vi "SubVI_HP4263A_1kHz.vi"(4 "error in (no error)":errorcluster, 5 "averaging count (1)":i16=1 min=1 max=256 step=1, 6 "function (Z - Angle:0)":u16(ring) items=["Z - Angle", "R - X", "Y - Angle", "G - B", "CP - D", "CP - Q", "CP - G", "CS - D", "CS - Q", "CS - RS", "LP - D", "LP - Q", "LP - G", "LS - D", "LS - Q", "LS - RS", "LS - DCR (option 001 only)", "LP - DCR (option 001 only)", "L2 - N (option 001 only)", "L2 - M (option 001 only)", "L2 - R2 (option 001 only)"], 7 "VISA resource name":refnum<visa-resource-name>) -> (0 "error out":errorcluster, 1 "secondary reading":dbl format="%.5e", 2 "primary reading":dbl format="%.5e", 3 "status":u16)   [LabVIEW 2010]
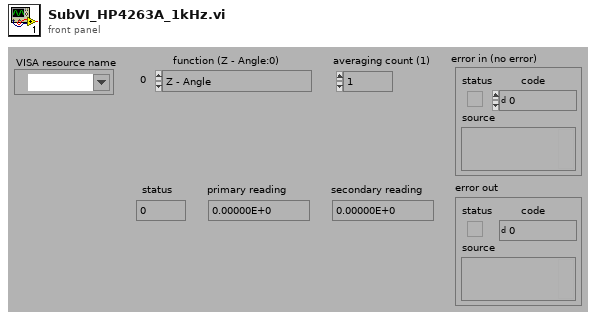
[diagram p1: front panel]
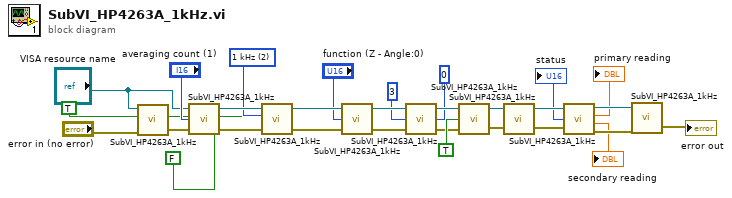
[diagram p0: block diagram]
diagram:
  w25 = u16 2 items=["100 Hz", "120 Hz", "1 kHz", "10 kHz", "20 kHz (option 002 ONLY)", "100 kHz"] ("frequency (100 Hz:0)")
  n1 = call "SubVI_HP4263A_1kHz.vi"("error in (no error)"="error in (no error)", "VISA resource name"="VISA resource name") -> ("error out"=w20:errorcluster)  [unwired: 2 in, 3 out]
  n2 = call "SubVI_HP4263A_1kHz.vi"("state (on:T)"=FALSE, "error in (no error)"=w20, "count (1)"="averaging count (1)", "VISA session"="VISA resource name") -> ("error out"=w28:errorcluster, "dup VISA session"=w26:refnum<visa-resource-name>)
  n3 = call "SubVI_HP4263A_1kHz.vi"("error in (no error)"=w28, "line frequency (60 Hz:F)"=TRUE, "frequency (100 Hz:0)"=w25, "VISA session"=w26) -> ("error out"=w29:errorcluster, "dup VISA session"=w27:refnum<visa-resource-name>)  [unwired: 1 in]
  n4 = call "SubVI_HP4263A_1kHz.vi"("error in (no error)"=w29, "function (Z - Angle:0)"="function (Z - Angle:0)", "VISA session"=w27) -> ("error out"=w9:errorcluster, "dup VISA session"=w8:refnum<visa-resource-name>)  [unwired: 1 in]
  n5 = call "SubVI_HP4263A_1kHz.vi"("trigger delay (sec)"=0, "error in (no error)"=w9, "trigger source (int:0)"=3, "VISA session"=w8) -> ("error out"=w13:errorcluster, "dup VISA session"=w14:refnum<visa-resource-name>)
  n6 = call "SubVI_HP4263A_1kHz.vi"("error in (no error)"=w13, "initiate mode (cont:T)"=TRUE, "VISA session"=w14) -> ("error out"=w16:errorcluster, "dup VISA session"=w15:refnum<visa-resource-name>)  [unwired: 1 in]
  n7 = call "SubVI_HP4263A_1kHz.vi"("error in (no error)"=w16, "VISA session"=w15) -> ("error out"=w11:errorcluster, "dup VISA session"=w12:refnum<visa-resource-name>)
  n8 = call "SubVI_HP4263A_1kHz.vi"("VISA session"=w12, "error in (no error)"=w11) -> ("status"=→"status":u16, "dup VISA session"=w22:refnum<visa-resource-name>, "primary reading"=→"primary reading":dbl, "secondary reading"=→"secondary reading":dbl, "error out"=w23:errorcluster)  [unwired: 2 out]
  n9 = call "SubVI_HP4263A_1kHz.vi"("error in (no error)"=w23, "dup VISA session"=w22) -> ("error out"=→"error out":errorcluster)  [unwired: 1 in]
